vi "Remove Endpoint Configuration.vi"(8 "error in (no error)":errorcluster, 10 "Endpoint":string, 11 "Endpoint Config Section Ref in":T1 format="%.0x") -> (0 "error out":errorcluster, 1 "Removed":bool, 3 "Endpoint Config Section Ref out":T1 format="%.0x")   [LabVIEW 2017, in "SLSC Switch Scripting.lvlib"]
uses:
  SLSC Switch Scripting.lvlib
  <vilib>/NI Veristand/Custom Device API/Custom Device Item Ref.ctl
  <vilib>/NI VeriStand/Custom Device API/Custom Device API.lvlib
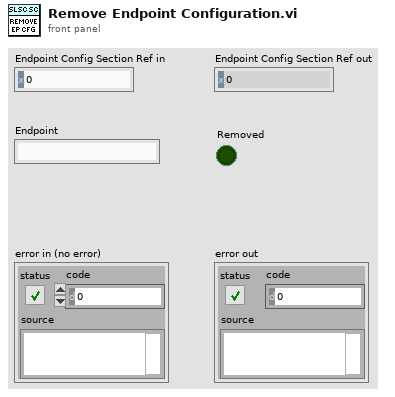
[diagram p1: front panel]
types:
  T1 = typedef "Custom Device API.lvlib/Custom Device Item Ref.ctl" = u64
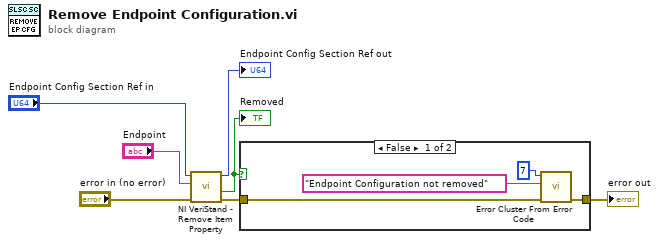
[diagram p0: block diagram]
diagram:
  n1 = call <vilib>:"NI VeriStand - Remove Item Property.vi"("error in (no error)"="error in (no error)", "Property Name"="Endpoint", "Item Ref in"="Endpoint Config Section Ref in") -> ("error out"=w2:errorcluster, "Removed"=w3:bool, "Item Ref out"=→"Endpoint Config Section Ref out":T1)  [unwired: 6 in]
  "Removed" <- w3
  n2 = case shown="False" w3 {
    tunnel: w2 -> [w9 w12]
    tunnel: [w8 w12] -> w1
    frame False {
      n3 = call <vilib>:"Error Cluster From Error Code.vi"("error in (no error)"=w9, "error message (\"\")"="Endpoint Configuration not removed" ("error message (\"\")"), "error code (0)"=7) -> ("error out"=w8:errorcluster)  [unwired: 6 in]
    }
    frame True {
    }
  }
  "error out" <- w1
